vi "ConfigureCurrent.vi"(8 "error in (no error)":errorcluster, 10 "Current(0)":dbl, 11 "VirtualPower in":refnum<class "VirtualPower.lvclass">) -> (0 "error out":errorcluster, 3 "VirtualPower out":refnum<class "VirtualPower.lvclass">)   [LabVIEW 2020, in "PowerControl.lvlib" / "VirtualPower.lvclass"]
uses:
  VirtualPower.lvclass
  VirtualPower.lvclass/VirtualPower.ctl
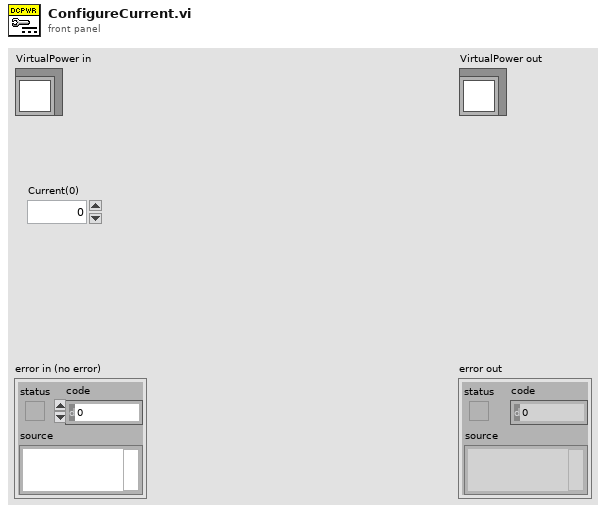
[diagram p1: front panel]
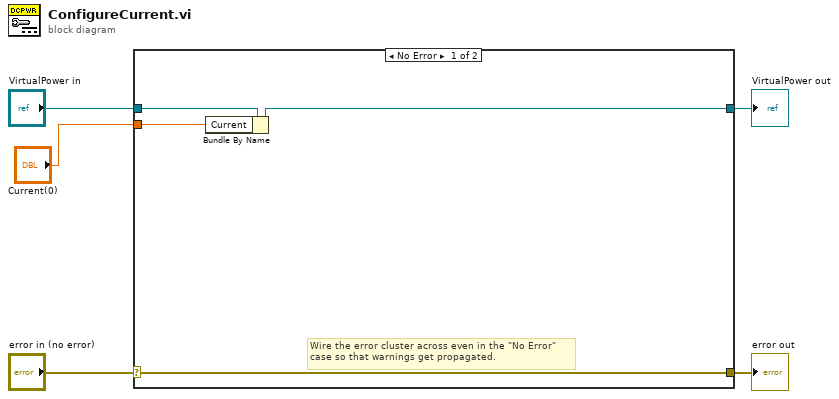
[diagram p0: block diagram]
diagram:
  n1 = case shown="No Error" "error in (no error)" {
    selector: "error in (no error)" -> [w8 w11]
    tunnel: [w8 w11] -> w4
    tunnel: [w7 w10] -> w2
    tunnel: "VirtualPower in" -> [w9 w10]
    tunnel: "Current(0)" -> [w6 _]
    frame No Error {
      # "Wire the error cluster across even in the \"No Error\"\ncase so that warnings get propagated."
      n2 = Bundle By Name(cluster=w9, "Current"=w6) -> (w7:refnum<class "VirtualPower.lvclass">)
    }
    frame Error {
    }
  }
  "error out" <- w4
  "VirtualPower out" <- w2
